vi "Generate Command String.vi"(0 "ITX Commands in":refnum<class "ITX Commands.lvclass">, 3 "error in (no error)":errorcluster) -> (7 "ITX Commands out":refnum<class "ITX Commands.lvclass">, 8 "ITX Commands":string, 10 "error out":errorcluster)   [LabVIEW 2016, in "ITX Commands.lvclass"]
uses:
  ITX Commands.lvclass
  ITX Commands.lvclass/ITX Commands.ctl
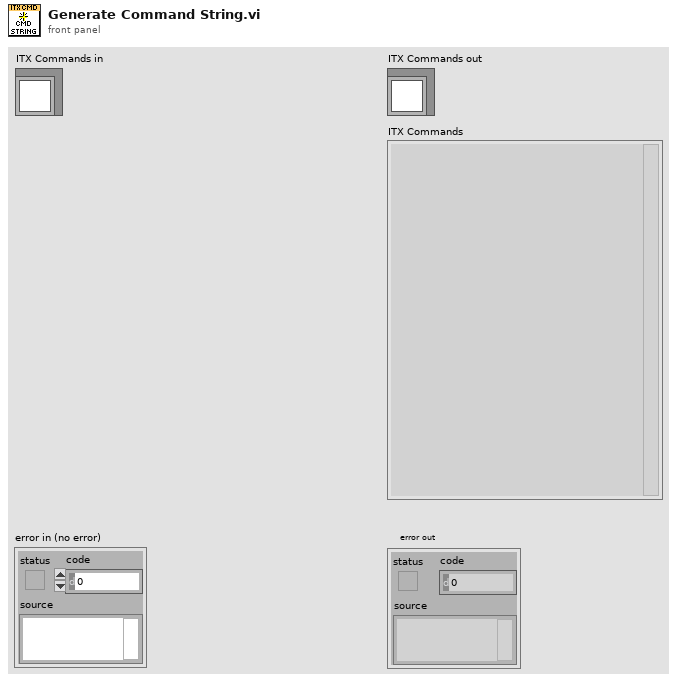
[diagram p1: front panel]
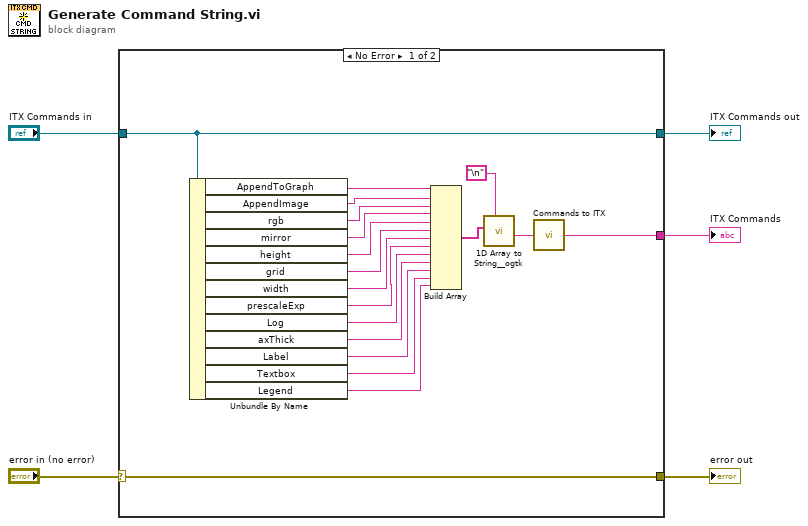
[diagram p0: block diagram]
diagram:
  n1 = case shown="No Error" "error in (no error)" {
    selector: "error in (no error)" -> [w24 w26]
    tunnel: [w24 w26] -> w4
    tunnel: [w7 w25] -> w2
    tunnel: "ITX Commands in" -> [w7 w25]
    tunnel: [w8 _] -> w1
    frame No Error {
      n2 = Unbundle By Name(w7) -> ("AppendToGraph"=w11:string, "AppendImage"=w12:string, "rgb"=w13:string, "mirror"=w14:string, "height"=w15:string, "grid"=w16:string, "width"=w17:string, "prescaleExp"=w18:string, "Log"=w19:string, "axThick"=w20:string, "Label"=w21:string, "Textbox"=w22:string, "Legend"=w6:string)
      n3 = Build Array(w11, w12, w13, w14, w15, w16, w17, w22, w18, w19, w20, w21, w6) -> (w23:string[])
      n4 = call <userlib>:"1D Array to String__ogtk.vi"("delimiter (Tab)"="\n", "Array of Strings"=w23) -> ("delimited string"=w9:string)  [unwired: 9 in]
      n5 = call "Commands to ITX.vi"("Commands"=w9) -> ("ITX Commands"=w8:string)
    }
    frame Error {
    }
  }
  "error out" <- w4
  "ITX Commands out" <- w2
  "ITX Commands" <- w1
